vi "PressureAndTimeSamples.vi"() -> ()   [LabVIEW 2012]
panel:
  in  "PressureAndTimeSamples":T1
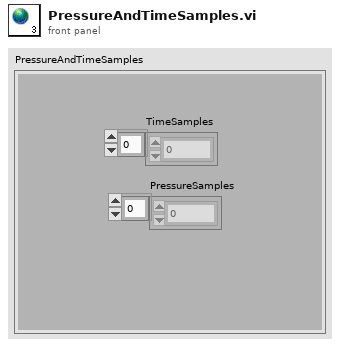
[diagram p1: front panel]
types:
  T1 = cluster{"TimeSamples":dbl[], "PressureSamples":dbl[]}
diagram:
